vi "Target.vi"() -> ()   [LabVIEW 2013]
uses:
  <vilib>/eio/EIONode/EIONode.xnode
  <vilib>/rvi/eio/common/nirviEmuTemplateMethod_errors.vi
  <vilib>/Platform/TimedLoop/XDataNode/XDataNode.xnode
  <vilib>/Platform/TimedLoop/XDataNode/timing_clust.ctl
  <vilib>/Platform/TimedLoop/XDataNode/XDNodeRunTimeDep.lvlib
  <vilib>/Platform/TimedLoop/XDataNode/wakeup.ctl
  <vilib>/Platform/TimedLoop/XDataNode/nitl_modes.ctl
panel:
  in  "3":u8=3
  out "Конец посылки?":bool
  in  "30":u8=30
  in  "40":u8=40
  in  "S_start":bool
  in  "SERDAT":bool[](array[boolean])=[TRUE, FALSE, FALSE, FALSE, TRUE, FALSE, FALSE, FALSE, TRUE, FALSE, FALSE, FALSE, FALSE, FALSE, FALSE, FALSE, FALSE, FALSE, FALSE, TRUE, FALSE, TRUE, TRUE, TRUE, TRUE, TRUE, TRUE, TRUE, TRUE, FALSE]
  out "TST":bool
  in  "RN":bool
  in  "Автомат":bool
  in  "Стоп":bool
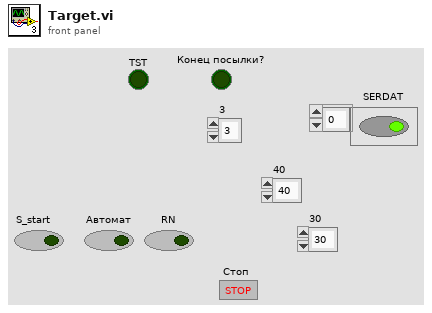
[diagram p1: front panel]
types:
  T1 = typedef "XDNodeRunTimeDep.lvlib/timing_clust.ctl" = cluster{"Expected End [f-1]":u64, "Actual End [f-1]":u64, "Finished Late? [f-1]":bool, "Expected End [i-1]":u64, "Actual End [i-1]":u64, "Finished Late? [i-1]":bool, "Expected Start [i]":u64, "Actual Start [i]":u64, "Expected Start [f]":u64, "Actual Start [f]":u64, "Source Name":string, "Structure Name":string, "Period":i64, "Deadline":i64, "Offset":i64, "Start":i64, "Priority":i32, "Timeout":i32, "Mode":T2, "Wakeup Reason":T3, "Error":errorcluster, "Source Type":string, "Secondary Source Type":string, "Global End Time":u64, "Global Start Time":u64, "Frame Duration":u64, "Iteration Duration":u64, "Assigned CPU":i32, "I/O Scan Engine Mode":u32}
  T2 = typedef "XDNodeRunTimeDep.lvlib/nitl_modes.ctl" = enum32{"No Change", "Process missed periods, maintain original phase", "Discard missed periods, maintain original phase", "Process missed periods, ignore original phase", "Discard missed periods, ignore original phase"}
  T3 = typedef "XDNodeRunTimeDep.lvlib/wakeup.ctl" = enum32{"Normal", "Aborted", "Asynchronous wakeup", "Timing source error", "Timed loop error", "Timeout"}
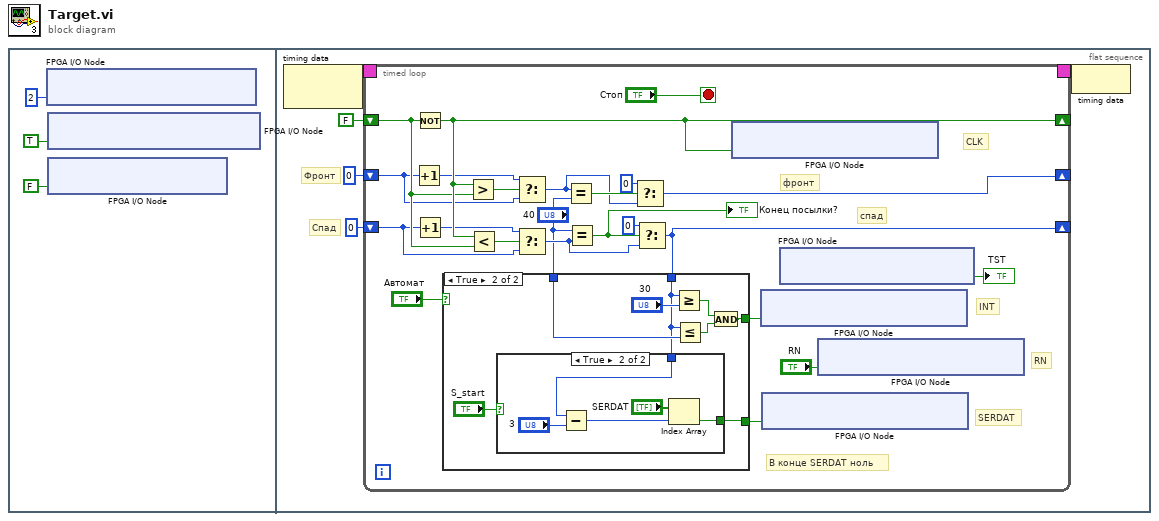
[diagram p0: block diagram]
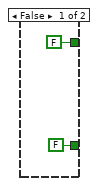
[diagram p2: hidden frame]
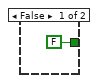
[diagram p3: hidden frame]
diagram:
  n1 = flat-sequence {
    frame #0 {
      n2 = xnode "FPGA I/O Node"("IO Module\\Local_Supply_Select"=u8 2 ("IO Module\\Local_Supply_Select")) -> ()  [unwired: 1 in, 1 out]
      n3 = xnode "FPGA I/O Node"("IO Module\\DDCA_DIO16-23_WE"=TRUE ("IO Module\\DDCA_DIO0-7_WE")) -> ()  [unwired: 1 in, 1 out]
      n4 = xnode "FPGA I/O Node"("IO Module\\DDCA_PFI_WE"=FALSE ("IO Module\\DDCA_PFI_WE")) -> ()  [unwired: 1 in, 1 out]
    }
    frame #1 {
      # "Спад"
      # "Фронт"
      n5 = node-c288() -> (w8:T1)  [unwired: 1 in]
      n6 = timed-loop {
        timing: w8 -> [_]
        timing-out: [_] -> w7
        shift-right: [w28] -> _
        shift-left: FALSE -> [w27]
        shift-right: [w10] -> _
        shift-left: u8 0 -> [w23]
        shift-right: [w13] -> _
        shift-left: u8 0 -> [w21]
        stop <- "Стоп" stop-if-true
        # "В конце SERDAT ноль"
        # "SERDAT"
        # "INT"
        # "спад"
        # "фронт"
        # "RN"
        # "CLK"
        n7 = Increment(x=w23) -> (x+1=w24:u8)
        n8 = Not(x=w27) -> (.not. x?=w28:bool)
        n9 = Increment(x=w21) -> (x+1=w22:u8)
        n10 = Greater?(x=w28, y=w27) -> (0:w26:bool)
        n11 = Less?(x=w28, y=w27) -> (x < y?=w25:bool)
        n12 = Select(t=w24, s=w26, f=w23) -> (s? t:f=w16:u8)
        n13 = Select(t=w22, s=w25, f=w21) -> (s? t:f=w17:u8)
        n14 = Equal?(x=w16, y="40") -> (x = y?=w20:bool)
        n15 = Equal?(x="40", y=w17) -> (x = y?=w9:bool)
        "Конец посылки?" <- w9
        n16 = Select(t=u8 0, s=w20, f=w16) -> (s? t:f=w10:u8)
        n17 = Select(t=u8 0, s=w9, f=w17) -> (s? t:f=w13:u8)
        n18 = case shown="True" "Автомат" {
          tunnel: [FALSE w37] -> w14
          tunnel: w13 -> [_ w35]
          tunnel: "40" -> [_ w39]
          tunnel: [FALSE w34] -> w11
          frame False {
          }
          frame True {
            n19 = case shown="True" "S_start" {
              tunnel: w35 -> [_ w47]
              tunnel: [FALSE ("Boolean") w43] -> w34
              frame False {
              }
              frame True {
                n20 = Subtract(x=w47, y="3") -> (x-y=w45:u8)
                n21 = Index Array(array="SERDAT", index=w45) -> (element=w43:bool)
              }
            }
            n22 = Greater Or Equal?(x=w35, y="30") -> (x >= y?=w40:bool)
            n23 = Less Or Equal?(x=w35, y=w39) -> (x <= y?=w38:bool)
            n24 = And(x=w40, y=w38) -> (x .and. y?=w37:bool)
          }
        }
        n25 = xnode "FPGA I/O Node"("IO Module\\DDCA_DIO17_Write"=w28) -> ()  [unwired: 1 in, 1 out]
        n26 = xnode "FPGA I/O Node"("IO Module\\DDCA_DIO19_Write"=w14) -> ()  [unwired: 1 in, 1 out]
        n27 = xnode "FPGA I/O Node"("IO Module\\DDCA_DIO23_Write"=w11) -> ()  [unwired: 1 in, 1 out]
        n28 = xnode "FPGA I/O Node"() -> ("IO Module\\DDCA_PFI2_Read"=→"TST":bool)  [unwired: 1 in, 1 out]
        n29 = xnode "FPGA I/O Node"("IO Module\\DDCA_DIO21_Write"="RN") -> ()  [unwired: 1 in, 1 out]
      }
      n30 = node-c288(w7) -> ()
    }
  }
